vi "Auto Fire Winch.vi"(11 "Run?":bool) -> (3 "Done":bool)   [LabVIEW 2013]
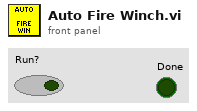
[diagram p1: front panel]
types:
  T1 = typedef "WPI_MotorControlDeviceRef.ctl" = cluster{"DeviceStatus":errorcluster, "Type":enum16{"PWM", "CAN"}, "PWM":cluster{"Digital Module":T2, "PWM Channel":T3, "DeadBand":T4}, "CAN":cluster{"Device Number":u8, "Control Mode":T5, "Semaphore":T6, "Max Vout":dbl}, "Invert":bool, "TransformRef":T7, "InvTransformRef":T7}
  T2 = typedef "FPGA_TypedefDigitalModule.ctl" = enum16{"Digital Module 1", "Digital Module 2"}
  T3 = typedef "FPGA_DIOPWMChannel.ctl" = enum8{"PWM 1", "PWM 2", "PWM 3", "PWM 4", "PWM 5", "PWM 6", "PWM 7", "PWM 8", "PWM 9", "PWM 10", "Invalid"}
  T4 = typedef "WPI_PWMDeadband.ctl" = cluster{"Name":string, "maxPositivePwm":i32, "minPositivePwm":i32, "centerPwm":i32, "maxNegativePwm":i32, "minNegativePwm":i32, "angularRange":u16}
  T5 = typedef "WPI_CANJaguar_ControlMode.ctl" = enum8{"Percent VBus", "Current", "Speed", "Position", "Voltage"}
  T6 = typedef "Semaphore RefNum" = refnum<k1>
  T7 = typedef "WPI_PWMTransform_ConPane.ctl" = refnum<vi>
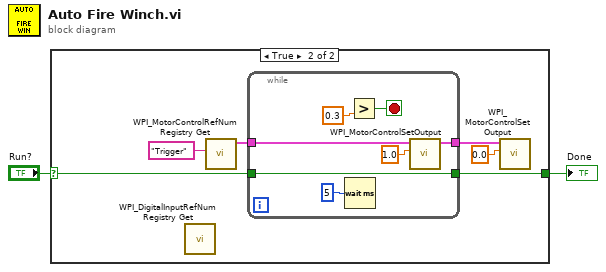
[diagram p0: block diagram]
diagram:
  n1 = case shown="True" "Run?" {
    selector: "Run?" -> [w3 w5]
    tunnel: [w3 w4] -> w1
    frame False {
    }
    frame True {
      n2 = call <vilib>:"WPI_DigitalInputRefNum Registry Get.vi"() -> ()  [unwired: 10 in, 2 out]
      n3 = call <vilib>:"WPI_MotorControlRefNum Registry Get.vi"("refnum name"="Trigger") -> ("MotorControlDevRef"=w7:T1)  [unwired: 9 in, 1 out]
      n4 = while {
        tunnel: w7 -> [w14]
        tunnel: [w15] -> w6
        tunnel: w5 -> [w11]
        tunnel: [w11] -> w4
        stop <- w12 stop-if-true
        n5 = Wait (ms)(milliseconds to wait=u32 5) -> ()  [unwired: 1 out]
        n6 = Greater?(y=0.3) -> (0:w12:bool)  [unwired: 1 in]
        n7 = call <vilib>:"WPI_MotorControlSetOutput.vi"("Output"=1.0, "MotorControlDevRef"=w14) -> ("MotorControlDevRef"=w15:T1)  [unwired: 7 in, 2 out]
      }
      n8 = call <vilib>:"WPI_MotorControlSetOutput.vi"("Output"=0.0, "MotorControlDevRef"=w6) -> ()  [unwired: 7 in, 3 out]
    }
  }
  "Done" <- w1
